vi "scaler.vi"(11 "Input":dbl) -> (3 "Output":u8)   [LabVIEW 2017]
uses:
  <vilib>/addons/control/pid/pid.llb/PID Percentage to EGU (DBL).vi
  <vilib>/addons/control/pid/NI_PID_pid.lvlib
panel:
  in  "Decay":dbl
  in  "Mode":enum16{"Color Organ"}(ring)
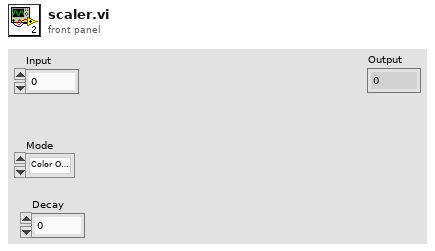
[diagram p1: front panel]
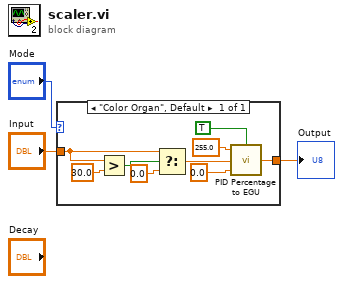
[diagram p0: block diagram]
diagram:
  n1 = case shown="\"Color Organ\", Default" "Mode" {
    tunnel: "Input" -> [w9]
    tunnel: [w5] -> w1
    frame "Color Organ", Default {
      n2 = Greater?(x=w9, y=30.0) -> (0:w11:bool)
      n3 = Select(t=w9, s=w11, f=0.0) -> (s? t:f=w8:dbl)
      n4 = call-poly <vilib>:"PID Percentage to EGU.vi"("coerce output to range? (T)"=TRUE, "minimum (EGU)"=0.0, "% span"=w8, "maximum (EGU)"=255.0) -> ("output (EGU)"=w5:dbl)
    }
  }
  "Output" <- w1
